vi "GetText.vi"(8 "error in":errorcluster, 11 "Daqmx Module editor node in":refnum<class "DAQmx Module Editor Node.lvclass">) -> (0 "error out":errorcluster, 1 "additional text":string, 2 "text":string, 3 "Daqmx Module editor node out":refnum<class "DAQmx Module Editor Node.lvclass">, 4 "glyph":string)   [LabVIEW 2014, in "DAQmx Module Editor Node.lvclass"]
doc: "Use this VI to display the name of the module in the tree and to specify the desired glyph in the configuration editor."
uses:
  DAQmx Module Editor Node.lvclass
  <vilib>/NI/DCAF/Tag Editor Core/Configuration Editor/Classes/Module editor node/Read display name.vi
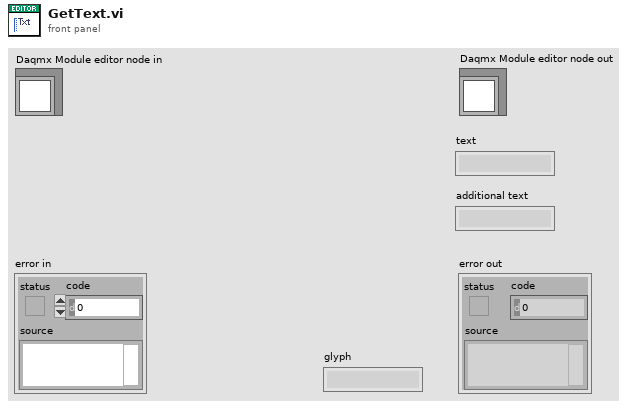
[diagram p1: front panel]
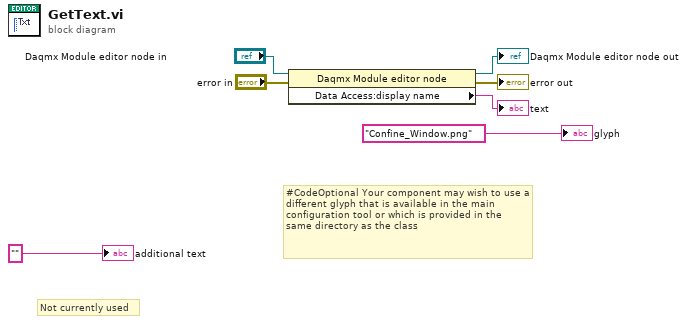
[diagram p0: block diagram]
diagram:
  # "Not currently used"
  # "#CodeOptional Your component may wish to use a different glyph that is available in the main configuration tool or which is provided in the same directory as the class"
  n1 = property class="Daqmx Module editor node"(reference="Daqmx Module editor node in", error in="error in") -> (reference out=→"Daqmx Module editor node out":refnum<class "DAQmx Module Editor Node.lvclass">, error out=→"error out":errorcluster, "Data Access:display name"=→"text":string)
  "additional text" <- "" ("additional text")
  "glyph" <- "Confine_Window.png" ("glyph")
